vi "ReadFIFODigitizer.vi"(4 "Read/nElement Count":bool=TRUE, 6 "Arm Trigger":bool=TRUE, 7 "range (V)":dbl=2.0, 8 "error in":errorcluster, 9 "Sample Rate":dbl=800000000.0 format="%#_13p", 10 "Number of Elements":u32, 11 "resource name":T1 caption="RIO Device") -> (0 "error out":errorcluster, 1 "Output Wave Int":u16[](array[numeric]), 2 "Elements Remaining":u32, 3 "Analog Output":waveform(ext)(graph)={"t0"=timestamp(0 s since 1904-01-01), "dt"=1.25e-09, "Y"=array[2048 elements]} caption="Acquired Waveform")   [LabVIEW 2018]
uses:
  <vilib>/userdefined/High Color/nirio_resource_hc.ctl
  <vilib>/Utility/error.llb/Error Cluster From Error Code.vi
  <vilib>/rvi/errors/niLvFpgaAdjustHostInterfaceError.vi
  <vilib>/FPGAPlugInAG/Dynamic/niLvFpga_Close_Dynamic.vi
  <vilib>/rvi/interface/nirviReadWriteControl/nirviReadWriteControl.xnode
  <vilib>/rvi/interface/nirviMethod/nirviMethod.xnode
  <vilib>/rvi/interface/nirviCloseFPGA/nirviCloseFPGA.xnode
  NiFpgaLv.dll
  <vilib>/rvi/interface/Simulation/niFpgaSimulationCallBeginRW.vi
  <vilib>/FPGAPlugInAG/Dynamic/niLvFpga_ReadFifo_Dynamic.vi
  <vilib>/rvi/errors/niLvFpgaMergeErrorWithErrorCode.vi
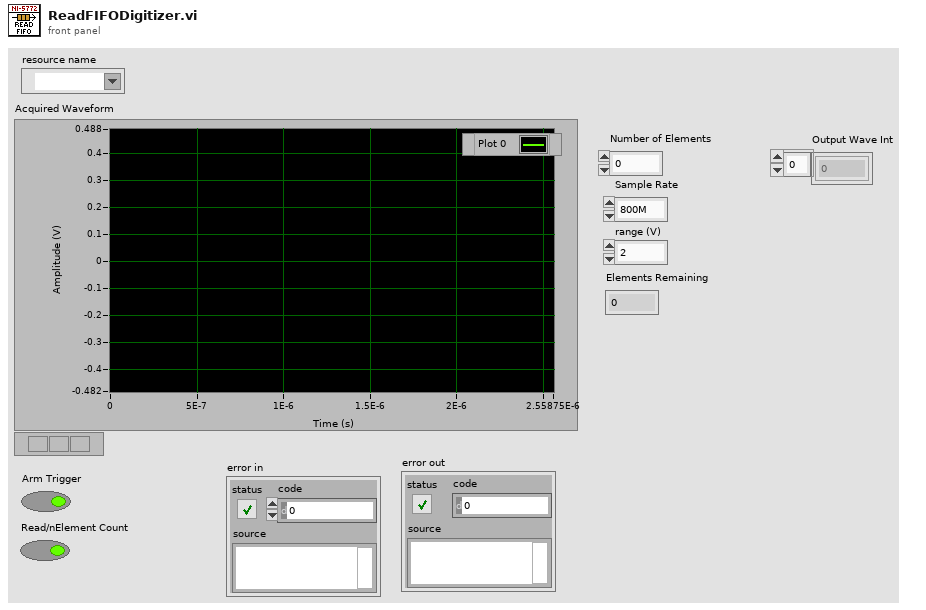
[diagram p1: front panel]
types:
  T1 = typedef "nirio_resource_hc.ctl" = tag
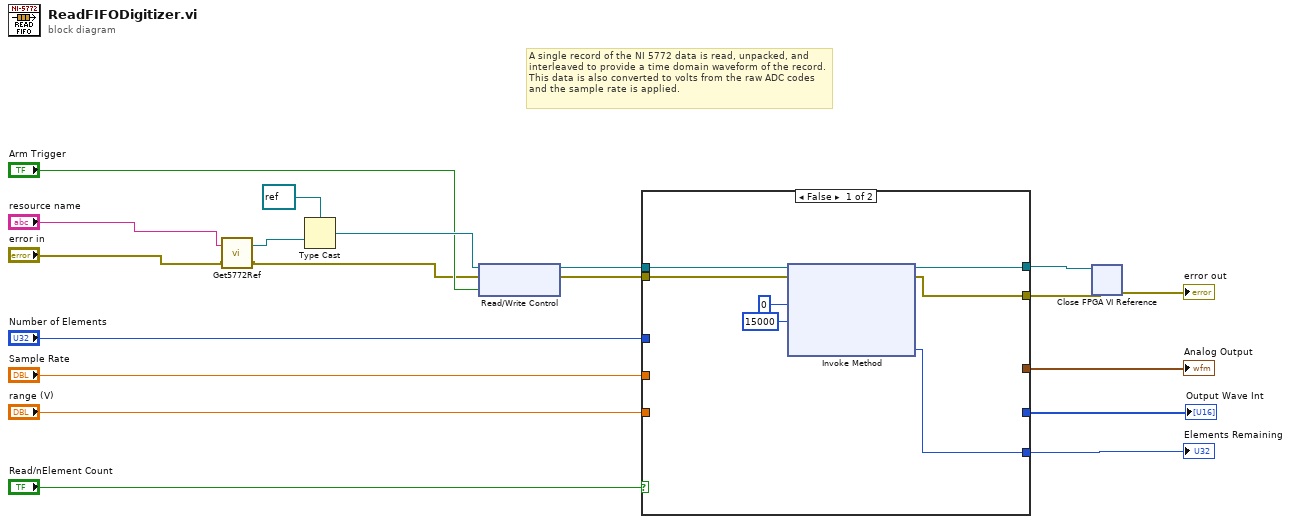
[diagram p0: block diagram]
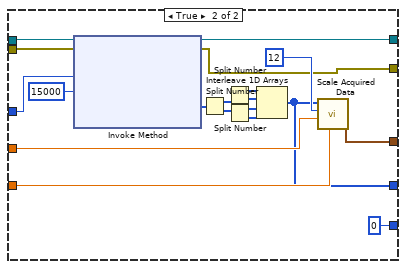
[diagram p2: hidden frame]
diagram:
  # "A single record of the NI 5772 data is read, unpacked, and interleaved to provide a time domain waveform of the record. This data is also converted to volts from the raw ADC codes and the sample rate is applied."
  n1 = call "Get5772Ref.vi"("error in (no error)"="error in", "RIO Device IN"="resource name") -> ("error out"=w4:errorcluster, "FPGA VI Reference Out"=w3:refnum<k20>)
  n2 = Type Cast(type=refnum<k20> refnum ("FPGA VI Reference Out"), x=w3) -> (*(type *) &x=w14:refnum<k20>)
  n3 = xnode "Read/Write Control"("FPGA VI Reference In"=w14, "error in"=w4, "Arm Trigger"="Arm Trigger") -> ("FPGA VI Reference Out"=w19:refnum<k20>, "error out"=w18:errorcluster)
  n4 = case shown="False" "Read/nElement Count" {
    tunnel: w19 -> [w26 w45]
    tunnel: w18 -> [w25 w44]
    tunnel: "Sample Rate" -> [_ w42]
    tunnel: "range (V)" -> [_ w34]
    tunnel: [_ w33] -> w15
    tunnel: "Number of Elements" -> [_ w32]
    tunnel: [w23 w31] -> w8
    tunnel: [w22 w30] -> w7
    tunnel: [w21 u32 0 ("Elements Remaining")] -> w9
    tunnel: [_ w28] -> w1
    frame False {
      n5 = xnode "Invoke Method"("FPGA VI Reference In"=w26, "error in"=w25, "Number of Elements"=u32 0, "Timeout (ms)"=15000) -> ("FPGA VI Reference Out"=w23:refnum<k20>, "error out"=w22:errorcluster, "Elements Remaining"=w21:u32)  [unwired: 1 out]
    }
    frame True {
      n6 = xnode "Invoke Method"("FPGA VI Reference In"=w45, "error in"=w44, "Number of Elements"=w32, "Timeout (ms)"=15000) -> ("FPGA VI Reference Out"=w31:refnum<k20>, "error out"=w30:errorcluster, "Data"=w41:u64[])  [unwired: 1 out]
      n7 = Split Number(x=w41) -> (hi(x)=w40:u32[], lo(x)=w39:u32[])
      n8 = Split Number(x=w40) -> (hi(x)=w38:u16[], lo(x)=w35:u16[])
      n9 = Split Number(x=w39) -> (hi(x)=w36:u16[], lo(x)=w37:u16[])
      n10 = Interleave 1D Arrays(w38, w35, w36, w37) -> (w28:u16[])
      n11 = call "Scale Acquired Data.vi"("range (V)"=w34, "Sample Rate"=w42, "Number of Bits"=i16 12, "Data In"=w28) -> ("output waveform"=w33:waveform(ext))  [unwired: 7 out]
    }
  }
  "Analog Output" <- w15
  "Elements Remaining" <- w9
  "Output Wave Int" <- w1
  n12 = xnode "Close FPGA VI Reference"("FPGA VI Reference In"=w8, "error in"=w7) -> ("error out"=→"error out":errorcluster)
